vi "VI Methods - Row 2.vi"(7 "Format Options":T1={"Background"={"Public Scope"={"Option"=FALSE, "Color"=0, "Operator"=FALSE}, "Protected Scope"={"Option"=FALSE, "Color"=0, "Operator"=FALSE}, "Community Scope"={"Option"=FALSE, "Color"=0, "Operator"=FALSE}, "Private Scope"={"Option"=FALSE, "Color"=0, "Operator"=FALSE}, "Unknown Scope"={"Option"=FALSE, "Color"=0, "Operator"=FALSE}, "Auto Error Handling"={"Option"=FALSE, "Color"=0, "Operator"=FALSE}, "Inline"={"Option"=FALSE, "Color"=0, "Operator"=FALSE}, "Separate CC"={"Option"=FALSE, "Color"=0, "Operator"=FALSE}, "Execution Priority Normal"={"Option"=FALSE, "Color"=0, "Operator"=FALSE}, "Reentrancy Non-RE"={"Option"=FALSE, "Color"=0, "Operator"=FALSE}}, "Bookmark Options"={"Bookmarks as New Line in VI Descriptions"=TRUE, "Unique Bookmark Tags Only"=TRUE, "Include Tag and Text"=TRUE}}, 8 "Error in":errorcluster caption="Error in (no error)", 11 "VI Info":T4 caption="cluster") -> (0 "Error out":errorcluster, 1 "Column Headers":string[](array[string])=["Name", "Reentrant", "Inline", "Auto Error", "Compiled"], 3 "Table Row Text":string)   [LabVIEW 2023, in "VIDoc Printer - Confluence.lvlib" / "VIDoc Printer - Confluence.lvclass"]
uses:
  VIDoc Printer - Confluence.lvclass
  Parsing/TypeDefs/Method Spec Cluster.ctl
  Parsing/TypeDefs/VI Type Extended Enum.ctl
  <vilib>/picture/picture.llb/imagedata.ctl
  Parsing/TypeDefs/Class Dispatch Type Enum.ctl
  Parsing/TypeDefs/Controls Info Cluster.ctl
  <vilib>/Utility/miscctls.llb/LVKeyTypeDef.ctl
  <vilib>/Utility/miscctls.llb/LVPointTypeDef.ctl
  Parsing/SubVIs/Structure Reporter/Tree Cluster.ctl
  Settings/Printer Settings/Formatting Options.ctl
  Settings/Printer Settings/Background Formatting Cluster.ctl
  Settings/Printer Settings/Bookmark Options.ctl
  Confluence Formatting/Types/Text Alignment Combo Box.ctl
  VIDoc Printer - Confluence.lvclass/VIDoc Printer - Confluence.ctl
  Confluence Formatting/Confluence Formatting.lvlib
  Printer/VIDoc Printer.lvclass
  Parsing/VIDoc Parsing.lvlib
  Settings/Printer Settings/Printer Settings.lvclass
  Parsing/SubVIs/Structure Reporter/Structure Reporter.lvlib
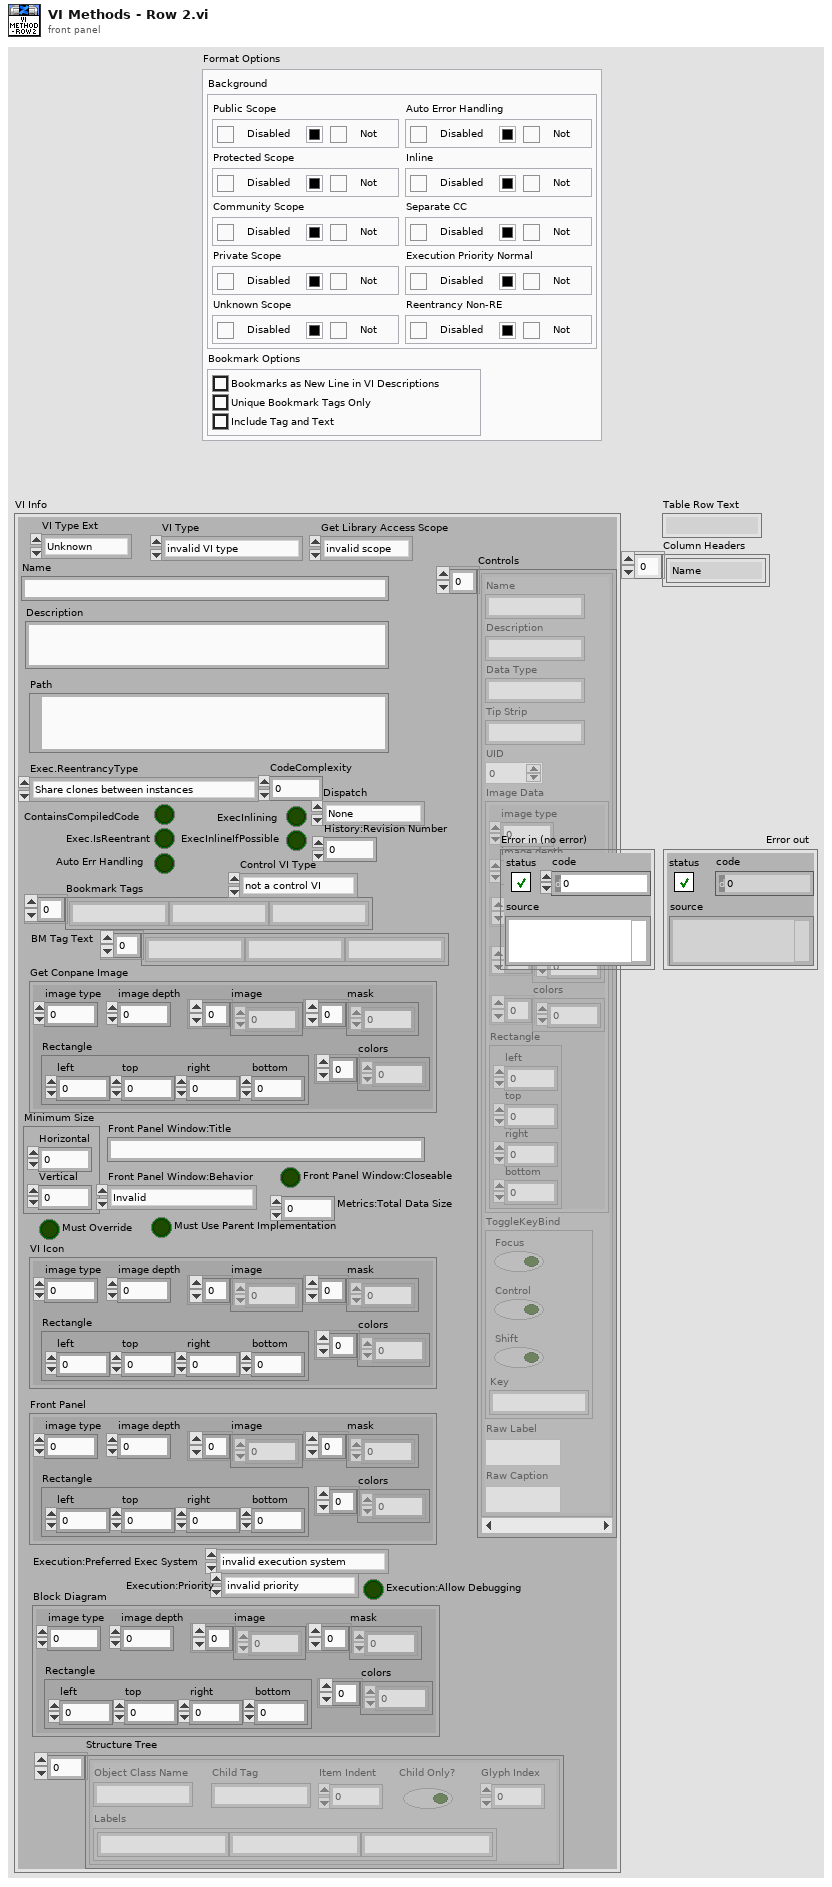
[diagram p1: front panel]
types:
  T1 = typedef "VIDoc Printer.lvlib/Printer Settings.lvclass/Formatting Options.ctl" = cluster{"Background":cluster{"Public Scope":T2, "Protected Scope":T2, "Community Scope":T2, "Private Scope":T2, "Unknown Scope":T2, "Auto Error Handling":T2, "Inline":T2, "Separate CC":T2, "Execution Priority Normal":T2, "Reentrancy Non-RE":T2}, "Bookmark Options":T3}
  T2 = typedef "VIDoc Printer.lvlib/Printer Settings.lvclass/Background Formatting Cluster.ctl" = cluster{"Option":bool, "Color":u32, "Operator":bool}
  T3 = typedef "VIDoc Printer.lvlib/Printer Settings.lvclass/Bookmark Options.ctl" = cluster{"Bookmarks as New Line in VI Descriptions":bool, "Unique Bookmark Tags Only":bool, "Include Tag and Text":bool}
  T4 = typedef "VIDoc Parsing.lvlib/Method Spec Cluster.ctl" = cluster{"VI Type Ext":T5, "Name":string, "Path":path, "Get Conpane Image":T6, "Description":string, "Get Library Access Scope":enum32{"invalid scope", "public", "private", "protected", "community"}, "Dispatch":T7, "ContainsCompiledCode":bool, "Exec.IsReentrant":bool, "Exec.ReentrancyType":enum16{"Share clones between instances", "Preallocate clone for each instance"}, "ExecInlining":bool, "ExecInlineIfPossible":bool, "Auto Err Handling":bool, "CodeComplexity":sgl, "Bookmark Tags":string[], "Control VI Type":enum32{"not a control VI", "control", "typedef", "strict typedef"}, "Controls":T8[], "VI Type":enum32{"invalid VI type", "Standard VI", "Control VI", "Global VI", "Polymorphic VI", "Configuration VI", "SubSystem", "Facade VI", "Method VI", "Statechart Diagram VI"}, "Minimum Size":T10, "Front Panel Window:Title":string, "Front Panel Window:Behavior":enum32{"Invalid", "Default", "Floating", "Floating/Auto-Hide", "Modal"}, "Front Panel Window:Closeable":bool, "Must Override":bool, "Must Use Parent Implementation":bool, "VI Icon":T6, "Front Panel":T6, "History:Revision Number":u32, "Metrics:Total Data Size":u32, "Execution:Allow Debugging":bool, "Execution:Preferred Exec System":enum32{"invalid execution system", "user interface", "standard", "instrument i/o", "data acquisition", "other 1", "other 2", "same as caller"}, "Execution:Priority":enum32{"invalid priority", "background priority", "normal priority", "above normal priority", "high priority", "time critical priority", "subroutine"}, "BM Tag Text":string[], "Block Diagram":T6, "Structure Tree":T11[]}
  T5 = typedef "VIDoc Parsing.lvlib/VI Type Extended Enum.ctl" = enum16{"Unknown", "Class Method", "Class Accessor Get", "Class Accessor Set", "Class Control", "Library Method", "Library Control", "VI", "Control"}
  T6 = typedef "imagedata.ctl" = cluster{"image type":i32, "image depth":i32, "image":u8[], "mask":u8[], "colors":u32[], "Rectangle":cluster{"left":i16, "top":i16, "right":i16, "bottom":i16}}
  T7 = typedef "VIDoc Parsing.lvlib/Class Dispatch Type Enum.ctl" = enum16{"None", "Static", "Dynamic"}
  T8 = typedef "VIDoc Parsing.lvlib/Controls Info Cluster.ctl" = cluster{"Name":string, "Description":string, "Data Type":string, "Tip Strip":string, "UID":i32, "Image Data":T6, "ToggleKeyBind":T9, "Raw Label":string, "Raw Caption":string}
  T9 = typedef "LVKeyTypeDef.ctl" = cluster{"Focus":bool, "Control":bool, "Shift":bool, "Key":string}
  T10 = typedef "LVPointTypeDef.ctl" = cluster{"Horizontal":i16, "Vertical":i16}
  T11 = typedef "VIDoc Parsing.lvlib/Structure Reporter.lvlib/Tree Cluster.ctl" = cluster{"Object Class Name":string, "Labels":string[], "Child Tag":string, "Item Indent":i32, "Child Only?":bool, "Glyph Index":i32}
  T12 = typedef "Confluence Formatting.lvlib/Text Alignment Combo Box.ctl" = string
  T13 = enum32{"invalid priority", "background priority", "normal priority", "above normal priority", "high priority", "time critical priority", "subroutine"}
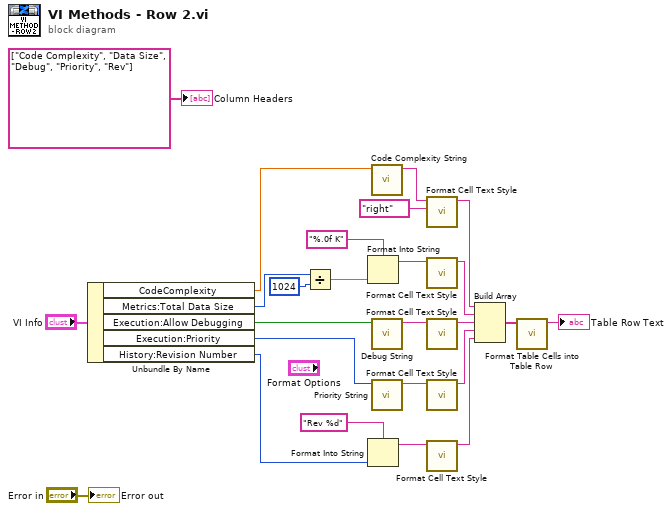
[diagram p0: block diagram]
diagram:
  n1 = Unbundle By Name("VI Info") -> ("CodeComplexity"=w15:sgl, "Metrics:Total Data Size"=w9:u32, "Execution:Allow Debugging"=w7:bool, "Execution:Priority"=w5:T13, "History:Revision Number"=w2:u32)
  n2 = Divide(x=w9, y=u32 1024) -> (x/y=w10:dbl)
  n3 = Format Into String(format string="%.0f K", w10) -> (resulting string=w8:string)  [unwired: 2 in, 1 out]
  n4 = Format Into String(format string="Rev %d", w2) -> (resulting string=w1:string)  [unwired: 2 in, 1 out]
  n5 = call "Code Complexity String.vi"("CodeComplexity"=w15) -> ("Code Complexity String"=w14:string)  [unwired: 10 in]
  n6 = call "Debug String.vi"("Allow Debugging"=w7) -> ("Debug String"=w6:string)  [unwired: 10 in]
  n7 = call "Priority String.vi"("Execution:Priority"=w5) -> ("Priority String"=w4:string)  [unwired: 10 in]
  n8 = call "Format Cell Text Style.vi"("Text Alignment (Left)"=T12 "right", "String"=w14) -> ("Formatted Text"=w18:string)  [unwired: 8 in, 1 out]
  n9 = call "Format Cell Text Style.vi"("String"=w8) -> ("Formatted Text"=w22:string)  [unwired: 9 in, 1 out]
  n10 = call "Format Cell Text Style.vi"("String"=w6) -> ("Formatted Text"=w23:string)  [unwired: 9 in, 1 out]
  n11 = call "Format Cell Text Style.vi"("String"=w4) -> ("Formatted Text"=w24:string)  [unwired: 9 in, 1 out]
  n12 = call "Format Cell Text Style.vi"("String"=w1) -> ("Formatted Text"=w25:string)  [unwired: 9 in, 1 out]
  n13 = Build Array(w18, w22, w23, w24, w25) -> (w19:string[])
  n14 = call "Format Table Cells into Table Row.vi"("Table Cells"=w19) -> ("Table Row Text"=→"Table Row Text":string)  [unwired: 10 in]
  "Error out" <- "Error in"
  "Column Headers" <- string[] ["Code Complexity", "Data Size", "Debug", "Priority", "Rev"]
